vi "InitializeDevice.vi"(8 "error in (no error)":errorcluster, 11 "NISTSimulation in":refnum<class "Simulation.lvclass">) -> (0 "error out":errorcluster, 3 "NISTSimulation out":refnum<class "Simulation.lvclass">)   [LabVIEW 2014, in "SamplerPlugins.lvlib" / "Simulation.lvclass"]
uses:
  Simulation.lvclass
  Simulation.lvclass/Simulation.ctl
  Accessors/Write EvtSignalArray.vi
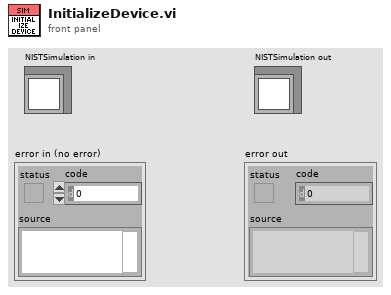
[diagram p1: front panel]
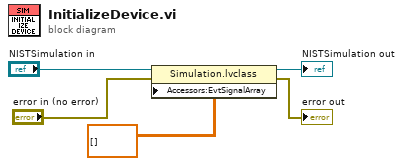
[diagram p0: block diagram]
diagram:
  n1 = property class="Simulation.lvclass"(reference="NISTSimulation in", error in="error in (no error)", "Accessors:EvtSignalArray"=dbl[][] [] ("EvtSignalArray")) -> (reference out=→"NISTSimulation out":refnum<class "Simulation.lvclass">, error out=→"error out":errorcluster)
